vi "Autonomous Sensor Read.vi"(11 "Sensor References":T1) -> (3 "Sensor Values":T5)   [LabVIEW 2013]
uses:
  Autonomous Sensor Values.ctl
  Autonomous Sensor References.ctl
  <vilib>/Rock Robotics/WPI/DigitalInput/WPI_DigitalInputDevRef.ctl
  <vilib>/Rock Robotics/SystemInterfaces/DIO/FPGA_DIOChannel.ctl
  <vilib>/Rock Robotics/SystemInterfaces/Typedef/FPGA_TypedefDigitalModule.ctl
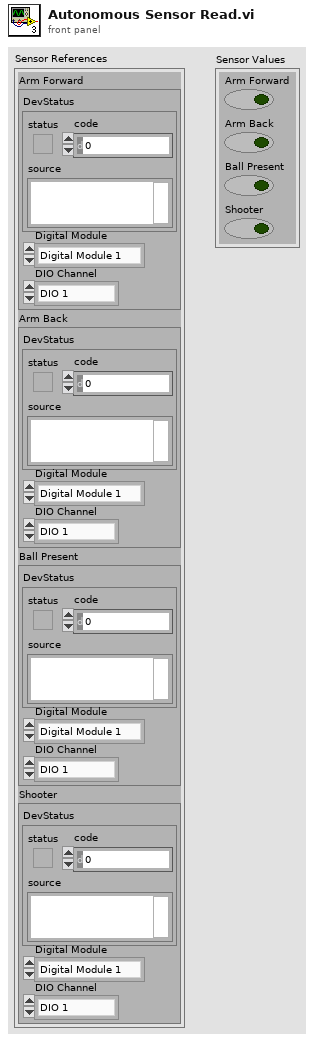
[diagram p1: front panel]
types:
  T1 = typedef "Autonomous Sensor References.ctl" = cluster{"Arm Forward":T2, "Arm Back":T2, "Ball Present":T2, "Shooter":T2}
  T2 = typedef "WPI_DigitalInputDevRef.ctl" = cluster{"DevStatus":errorcluster, "DIO Channel":T3, "Digital Module":T4}
  T3 = typedef "FPGA_DIOChannel.ctl" = enum8{"DIO 1", "DIO 2", "DIO 3", "DIO 4", "DIO 5", "DIO 6", "DIO 7", "DIO 8", "DIO 9", "DIO 10", "DIO 11", "DIO 12", "DIO 13", "DIO 14", "Invalid"}
  T4 = typedef "FPGA_TypedefDigitalModule.ctl" = enum16{"Digital Module 1", "Digital Module 2"}
  T5 = typedef "Autonomous Sensor Values.ctl" = cluster{"Arm Forward":bool, "Arm Back":bool, "Ball Present":bool, "Shooter":bool}
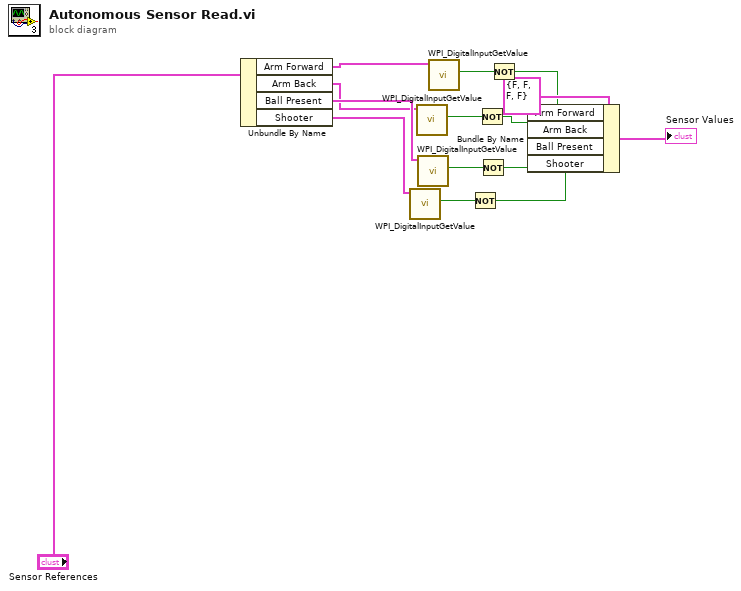
[diagram p0: block diagram]
diagram:
  n1 = Unbundle By Name("Sensor References") -> ("Arm Forward"=w3:T2, "Arm Back"=w7:T2, "Ball Present"=w8:T2, "Shooter"=w9:T2)
  n2 = call <vilib>:"WPI_DigitalInputGetValue.vi"("DigitalInputDevRef"=w9) -> ("Value"=w6:bool)  [unwired: 8 in, 2 out]
  n3 = call <vilib>:"WPI_DigitalInputGetValue.vi"("DigitalInputDevRef"=w7) -> ("Value"=w4:bool)  [unwired: 8 in, 2 out]
  n4 = call <vilib>:"WPI_DigitalInputGetValue.vi"("DigitalInputDevRef"=w8) -> ("Value"=w5:bool)  [unwired: 8 in, 2 out]
  n5 = call <vilib>:"WPI_DigitalInputGetValue.vi"("DigitalInputDevRef"=w3) -> ("Value"=w2:bool)  [unwired: 8 in, 2 out]
  n6 = Not(x=w6) -> (.not. x?=w13:bool)
  n7 = Not(x=w4) -> (.not. x?=w11:bool)
  n8 = Not(x=w5) -> (.not. x?=w12:bool)
  n9 = Not(x=w2) -> (.not. x?=w10:bool)
  n10 = Bundle By Name(cluster=T5 {"Arm Forward"=FALSE, "Arm Back"=FALSE, "Ball Present"=FALSE, "Shooter"=FALSE}, "Arm Forward"=w10, "Arm Back"=w11, "Ball Present"=w12, "Shooter"=w13) -> (→"Sensor Values":T5)
